vi "Read password file.vi"(8 "error in (no error)":errorcluster, 11 "file path":path=path "E:/Projects/bruce/PART11 & DI TOOLKIT/passwords.log") -> (0 "error out":errorcluster={"status"=FALSE, "code"=0, "source"="Read File+ (string): Read File"}, 3 "Access Configuration":T1={"Max ID attempts"=3, "Max password attempts"=4, "Expiration enabled"=TRUE, "Expire days"=90, "User array"=[{"Active?"=TRUE, "User ID"="CTI", "Password"="CTI", "Name"="Mike", "Security level"=10, "Expired?"=FALSE, "Expire sec"=inf, "Locked?"=FALSE, "New?"=FALSE}], "Min password char"=0} {"User array"."Expire sec" format="%.2f"})   [LabVIEW 2013]
doc: "This vi reads the encoded passwords file to return the access configuration information for all users."
uses:
  User Access Type defs/All users access configuration cluster.ctl
  User Access Type defs/User access cluster array.ctl
  User Access Type defs/User access cluster.ctl
  User Access Type defs/Security level U8.ctl
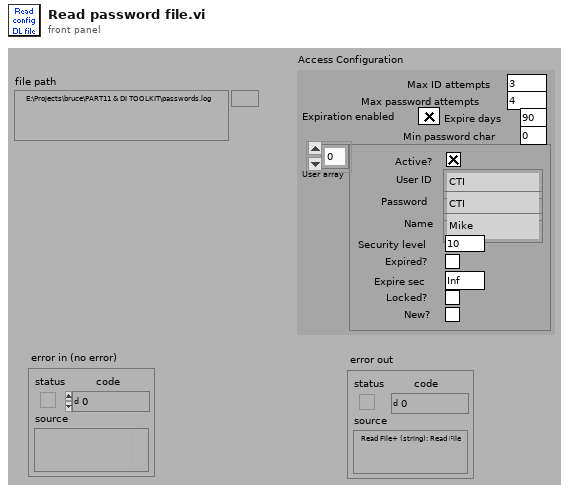
[diagram p1: front panel]
types:
  T1 = typedef "All users access configuration cluster.ctl" = cluster{"Max ID attempts":i32, "Max password attempts":i32, "Expiration enabled":bool, "Expire days":i32, "User array":T2, "Min password char":i32}
  T2 = typedef "User access cluster array.ctl" = T3[]
  T3 = typedef "User access cluster.ctl" = cluster{"Active?":bool, "User ID":string, "Password":string, "Name":string, "Security level":T4, "Expired?":bool, "Expire sec":dbl, "Locked?":bool, "New?":bool}
  T4 = typedef "Security level U8.ctl" = u8
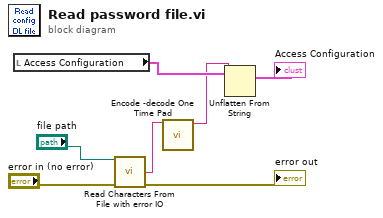
[diagram p0: block diagram]
diagram:
  n1 = local read "Access Configuration"() -> (w4:T1)
  n2 = call "Read Characters From File with error IO.vi"("file path (dialog if empty)"="file path", "error in (no error)"="error in (no error)") -> ("character string"=w2:string, "error out"=→"error out":errorcluster)  [unwired: 3 in, 9 out]
  n3 = call "Encode -decode One Time Pad.vi"("Text in"=w2) -> ("Text out"=w1:string)  [unwired: 2 in, 6 out]
  n4 = Unflatten From String(type=w4, binary string=w1) -> (value=→"Access Configuration":T1)  [unwired: 1 in, 4 out]
